vi "AutoscaleYaxis.vi"(8 "Has Coherence in plot?":bool, 10 "dB Range":dbl=40.0, 11 "WaveformGraph in":refnum<vi>) -> ()   [LabVIEW 2022 SP3]
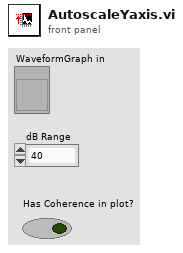
[diagram p1: front panel]
types:
  T1 = typedef "LVRangeTypeDef.ctl" = cluster{"Minimum":dbl, "Maximum":dbl, "Increment":dbl, "Minor Increment":dbl, "Start":dbl}
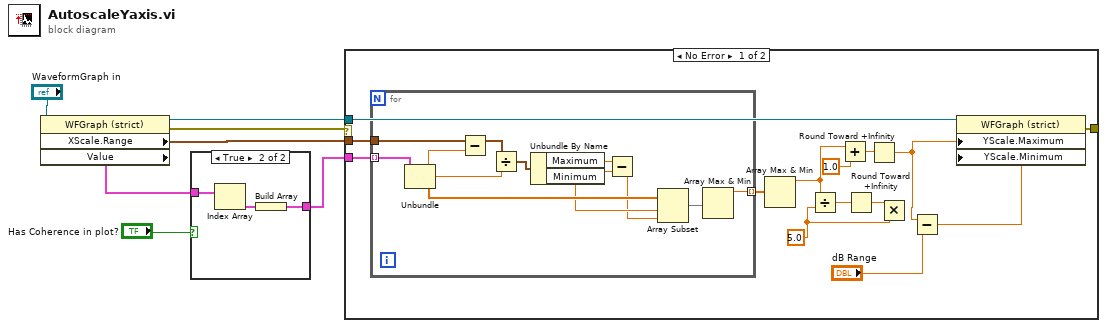
[diagram p0: block diagram]
diagram:
  n1 = property class="WFGraph (strict)"(reference="WaveformGraph in") -> (reference out=w5:refnum<vi>, error out=w4:errorcluster, "XScale.Range"=w6:T1, "Value"=w3:cluster{dbl, "df":dbl, dbl[]}[])  [unwired: 1 in]
  n2 = case shown="True" "Has Coherence in plot?" {
    tunnel: w3 -> [w8 w10]
    tunnel: [w8 w9] -> w2
    frame False {
    }
    frame True {
      n3 = Index Array(array=w10) -> (element=w11:cluster{dbl, "df":dbl, dbl[]})  [unwired: 1 in]
      n4 = Build Array(w11) -> (w9:cluster{dbl, "df":dbl, dbl[]}[])
    }
  }
  n5 = case shown="No Error" w4 {
    tunnel: w2 -> [w25 _]
    tunnel: w6 -> [w24 _]
    tunnel: w5 -> [w18 _]
    tunnel: [w12 _] -> _
    frame No Error {
      w21 = 5.0 ("y")
      n6 = for {
        tunnel: w25 -> [w26] mode=indexing
        tunnel: w24 -> [w36]
        tunnel: [w29] -> w17 mode=indexing
        n7 = Unbundle(w26) -> (w27:dbl, "df"=w37:dbl, w34:dbl[])
        n8 = Subtract(x=w36, y=w27) -> (x-y=w28:T1)
        n9 = Divide(x=w28, y=w37) -> (x/y=w35:T1)
        n10 = Unbundle By Name(w35) -> ("Maximum"=w33:dbl, "Minimum"=w32:dbl)
        n11 = Subtract(x=w33, y=w32) -> (x-y=w31:dbl)
        n12 = Array Subset(array=w34, index=w32, length=w31) -> (w30:dbl[])
        n13 = Array Max & Min(array=w30) -> (max value=w29:dbl)  [unwired: 3 out]
      }
      n14 = Array Max & Min(array=w17) -> (max value=w16:dbl)  [unwired: 3 out]
      n15 = Divide(x=w16, y=w21) -> (x/y=w23:dbl)
      n16 = Add(x=w16, y=1.0) -> (x+y=w14:dbl)
      n17 = Round Toward +Infinity(x=w23) -> (ceil(x): smallest int >= x=w22:dbl)
      n18 = Round Toward +Infinity(x=w14) -> (ceil(x): smallest int >= x=w13:dbl)
      n19 = Multiply(x=w22, y=w21) -> ()  [unwired: 1 out]
      n20 = Subtract(x=w13, y="dB Range") -> (x-y=w19:dbl)
      n21 = property class="WFGraph (strict)"(reference=w18, "YScale.Maximum"=w13, "YScale.Minimum"=w19) -> (error out=w12:errorcluster)  [unwired: 1 in, 1 out]
    }
    frame Error {
    }
  }
